vi "divide by 2.vi"(11 "Numeric in":dbl) -> (3 "Numeric out":dbl)   [LabVIEW 2020]
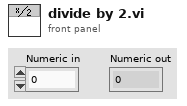
[diagram p1: front panel]
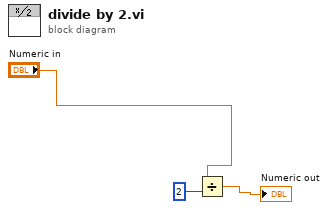
[diagram p0: block diagram]
diagram:
  n1 = Divide(x="Numeric in", y=2) -> (x/y=→"Numeric out":dbl)
